vi "ClassPanel.vi"(8 "error in (no error)":errorcluster caption="entrée d'erreur (pas d'erreur)", 11 "OR77200.lvclass":refnum<class "OR77200.lvclass">) -> (0 "error out":errorcluster caption="sortie d'erreur", 3 "OR77200.lvclass Out":refnum<class "OR77200.lvclass">)   [LabVIEW 2010, in "OR77200.lvclass"]
uses:
  OR77200.lvclass
  BaseDevice/BaseDevice.lvclass
panel:
  in  "SetActPos":bool
  in  "Acq":bool
  in  "Stop":bool
  out "Init Program":bool
  out "OR77200Mov":bool caption="SpexMov"
  in  "StopOR77200":bool caption="stopSpectro"
  in  "OR77200Pos":dbl=1000.0 caption="OR77200 (nm)" min=0.0 step=0.1 format="%#.1f"
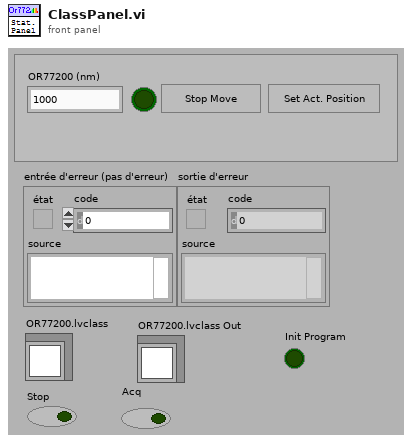
[diagram p1: front panel]
types:
  T1 = enum8{"Enabled", "Disabled", "Disabled and Grayed Out"}
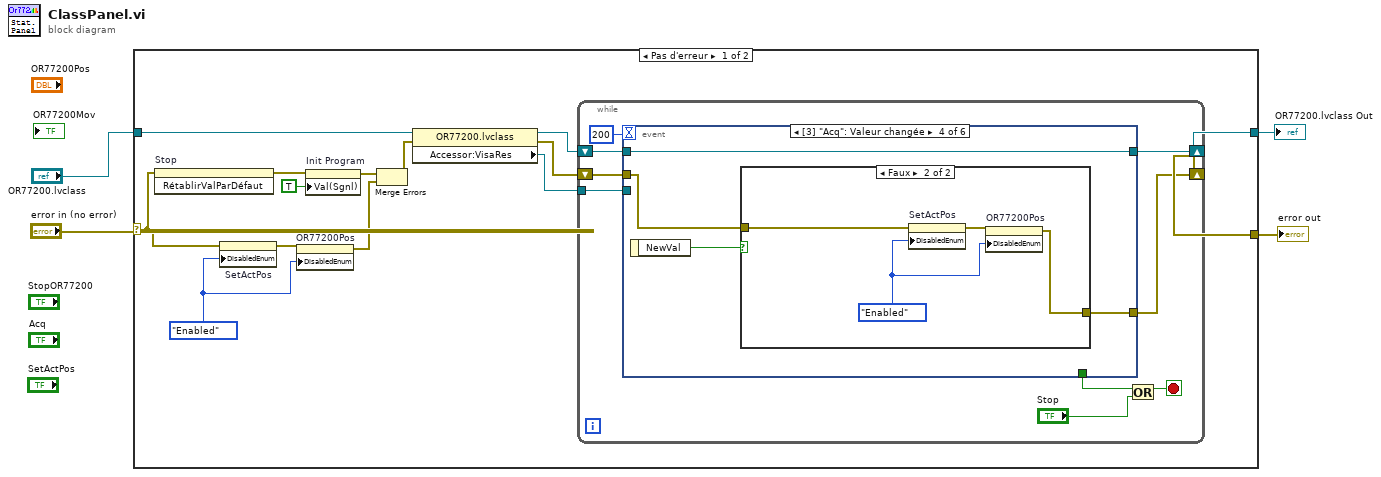
[diagram p0: block diagram]
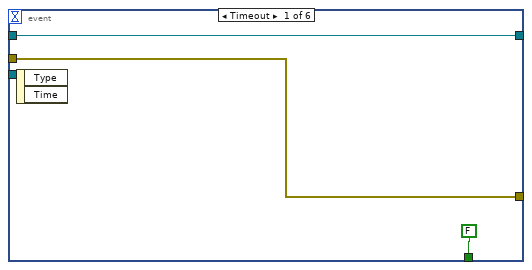
[diagram p2: hidden frame]
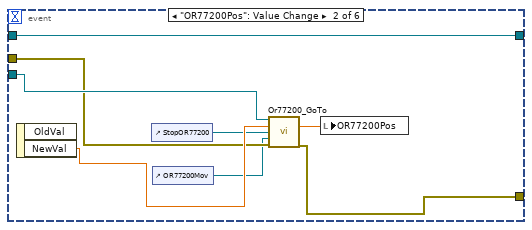
[diagram p3: hidden frame]
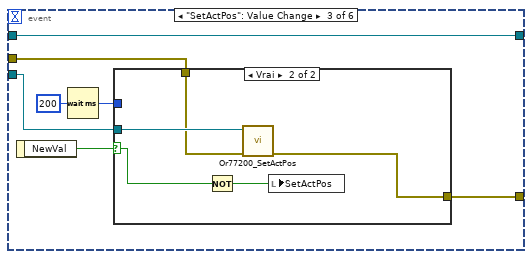
[diagram p4: hidden frame]
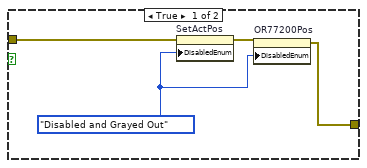
[diagram p6: hidden frame]
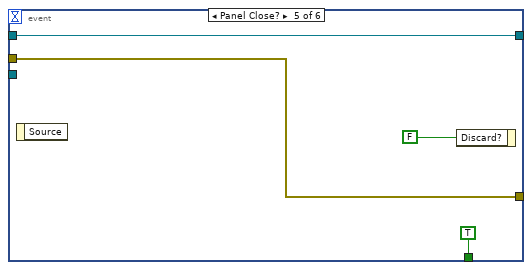
[diagram p7: hidden frame]
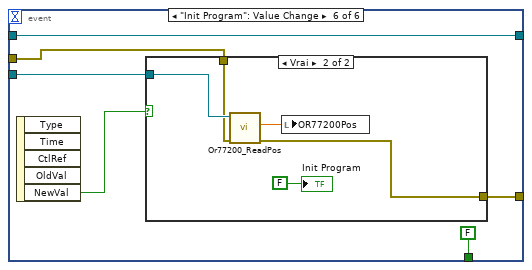
[diagram p8: hidden frame]
diagram:
  n1 = case shown="Pas d'erreur" "error in (no error)" {
    selector: "error in (no error)" -> [w7 w81]
    tunnel: [w18 w81] -> w3
    tunnel: "OR77200.lvclass" -> [w17 w80]
    tunnel: [w14 w80] -> w1
    frame No Error {
      w8 = T1."Enabled" ("Désactivé")
      n2 = invoke on="Stop" class="Bool (strict)" method="RétablirValParDéfaut"(error in=w7) -> (error out=w13:errorcluster)  [unwired: 2 in, 2 out]
      n3 = property on="SetActPos" class="Bool (strict)"(error in=w7, "DisabledEnum"=w8) -> (error out=w9:errorcluster)  [unwired: 1 in, 1 out]
      n4 = property on="OR77200Pos" class="NumDig (strict)"(error in=w9, "DisabledEnum"=w8) -> (error out=w5:errorcluster)  [unwired: 1 in, 1 out]
      n5 = property on="Init Program" class="Bool (strict)"(error in=w13, "Val(Sgnl)"=TRUE ("Valeur (Signalisation)")) -> (error out=w12:errorcluster)  [unwired: 1 in, 1 out]
      n6 = Merge Errors(w12, w5) -> (w6:errorcluster)
      n7 = property class="OR77200.lvclass"(reference=w17, error in=w6) -> (reference out=w10:refnum<class "OR77200.lvclass">, error out=w16:errorcluster, "Accessor:VisaRes"=w11:refnum<visa-resource-name>)
      n8 = while {
        shift-right: [w25] -> w18
        shift-left: w16 -> [w26]
        tunnel: w11 -> [w22]
        shift-right: [w21] -> w14
        shift-left: w10 -> [w24]
        stop <- w20 stop-if-true
        n9 = event shown="[3] \"Acq\": Valeur changée" {
          selector: _ -> [_ _ _ _ _ _]
          dyn-events: _ -> [_ _ _ _ _ _]
          timeout: 200 -> [_ _ _ _ _ _]
          tunnel: w26 -> [w28 w36 w41 w54 w65 w71]
          tunnel: [w28 w32 w40 w53 w65 w70] -> w25
          tunnel: w24 -> [w29 w31 w39 w52 w64 w69]
          tunnel: [FALSE _ _ _ TRUE FALSE] -> w23
          tunnel: [w29 w31 w39 w52 w64 w69] -> w21
          tunnel: w22 -> [_ w38 w42 _ _ w72]
          event Timeout {
            n10 = event-data() -> ()  [unwired: 1 in, 2 out]
          }
          event "OR77200Pos": Value Change {
            n11 = event-data() -> ("NewVal"=w37:dbl)  [unwired: 1 in, 1 out]
            n12 = control-ref of="StopOR77200"() -> (w35:refnum<vi>)
            n13 = control-ref of="OR77200Mov"() -> (w33:refnum<vi>)
            n14 = call <userlib>:"Or77200_GoTo.vi"("Port"=w38, "Lambda (nm)"=w37, "Stop Ref"=w35, "Move Ref"=w33, "error In"=w36) -> ("Lambda Out (nm)"=w34:dbl, "sortie d'erreur"=w32:errorcluster)  [unwired: 7 in, 2 out]
            n15 = local write "OR77200Pos"(w34) -> ()
          }
          event "SetActPos": Value Change {
            n16 = event-data() -> ("NewVal"=w45:bool)  [unwired: 1 in]
            n17 = Wait (ms)(milliseconds to wait=u32 200 ("attente (ms)")) -> (millisecond timer value=w44:u32)
            n18 = case shown="Vrai" w45 {
              selector: w45 -> [_ w51]
              tunnel: w44 -> [_ _]
              tunnel: w42 -> [_ w49]
              tunnel: w41 -> [w46 w48]
              tunnel: [w46 w47] -> w40
              frame False {
              }
              frame True {
                n19 = Not(x=w51) -> (.not. x?=w50:bool)
                n20 = call <userlib>:"Or77200_SetActPos.vi"("ErrorIn(No Error)"=w48, "Port"=w49) -> ("sortie d'erreur"=w47:errorcluster)  [unwired: 8 in, 1 out]
                n21 = local write "SetActPos"(w50) -> ()
              }
            }
          }
          event "Acq": Value Change {
            n22 = event-data() -> ("NewVal"=w55:bool)  [unwired: 1 in]
            n23 = case shown="Faux" w55 {
              tunnel: w54 -> [w59 w63]
              tunnel: [w56 w60] -> w53
              frame True {
                w58 = T1."Disabled and Grayed Out" ("Désactivé")
                n24 = property on="SetActPos" class="Bool (strict)"(error in=w59, "DisabledEnum"=w58) -> (error out=w57:errorcluster)  [unwired: 1 in, 1 out]
                n25 = property on="OR77200Pos" class="NumDig (strict)"(error in=w57, "DisabledEnum"=w58) -> (error out=w56:errorcluster)  [unwired: 1 in, 1 out]
              }
              frame False {
                w62 = T1."Enabled" ("Désactivé")
                n26 = property on="SetActPos" class="Bool (strict)"(error in=w63, "DisabledEnum"=w62) -> (error out=w61:errorcluster)  [unwired: 1 in, 1 out]
                n27 = property on="OR77200Pos" class="NumDig (strict)"(error in=w61, "DisabledEnum"=w62) -> (error out=w60:errorcluster)  [unwired: 1 in, 1 out]
              }
            }
          }
          event Panel Close? {
            n28 = event-data() -> ()  [unwired: 1 in, 1 out]
            n29 = event-data("Discard?"=FALSE ("Rejeter ?")) -> ()  [unwired: 1 in, 1 out]
          }
          event "Init Program": Value Change {
            n30 = event-data() -> ("NewVal"=w73:bool)  [unwired: 1 in, 4 out]
            n31 = case shown="Vrai" w73 {
              tunnel: w72 -> [_ w78]
              tunnel: w71 -> [w74 w76]
              tunnel: [w74 w75] -> w70
              frame False {
              }
              frame True {
                n32 = call <userlib>:"Or77200_ReadPos.vi"("error In"=w76, "Port"=w78) -> ("sortie d'erreur"=w75:errorcluster, "Lambda Out (nm)"=w77:dbl)  [unwired: 7 in, 1 out]
                n33 = local write "OR77200Pos"(w77) -> ()
                "Init Program" <- FALSE
              }
            }
          }
        }
        n34 = Or(x=w23, y="Stop") -> (x .or. y?=w20:bool)
      }
    }
    frame Error {
    }
  }
  "error out" <- w3
  "OR77200.lvclass Out" <- w1
